vi "update_zc_info2A.vi"(0 "ywxinxi":string, 4 "didian":string, 5 "ruku":string, 6 "number":string, 7 "lingyong":string, 8 "syren":string, 9 "zrren":string, 10 "zrbumen":string) -> (1 "data_str":string)   [LabVIEW 2017, in "Lib_code.lvlib"]
uses:
  Lib_code.lvlib
panel:
  out "error":errorcluster caption="error out 4"
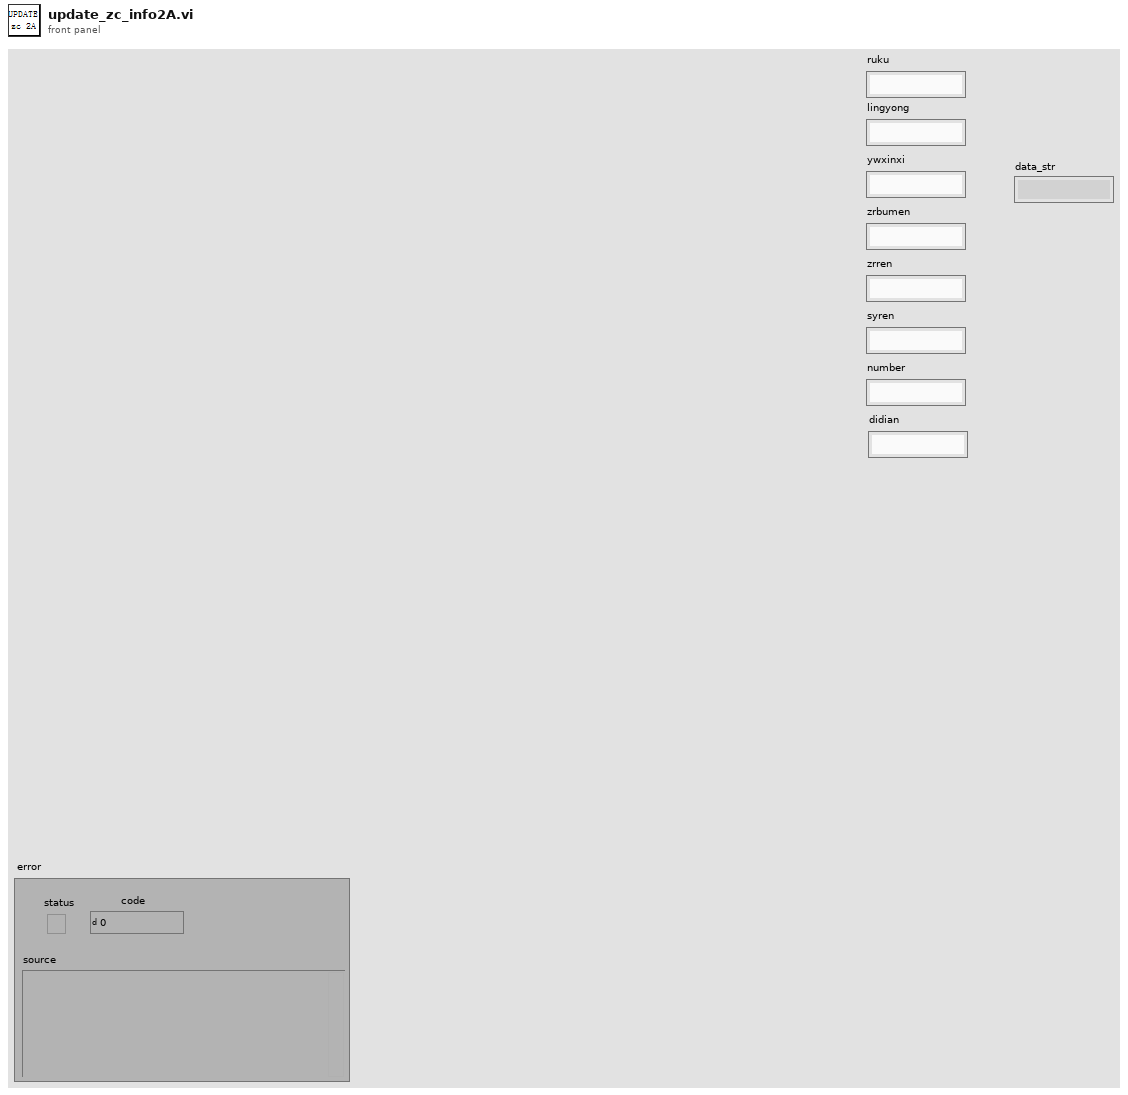
[diagram p1: front panel]
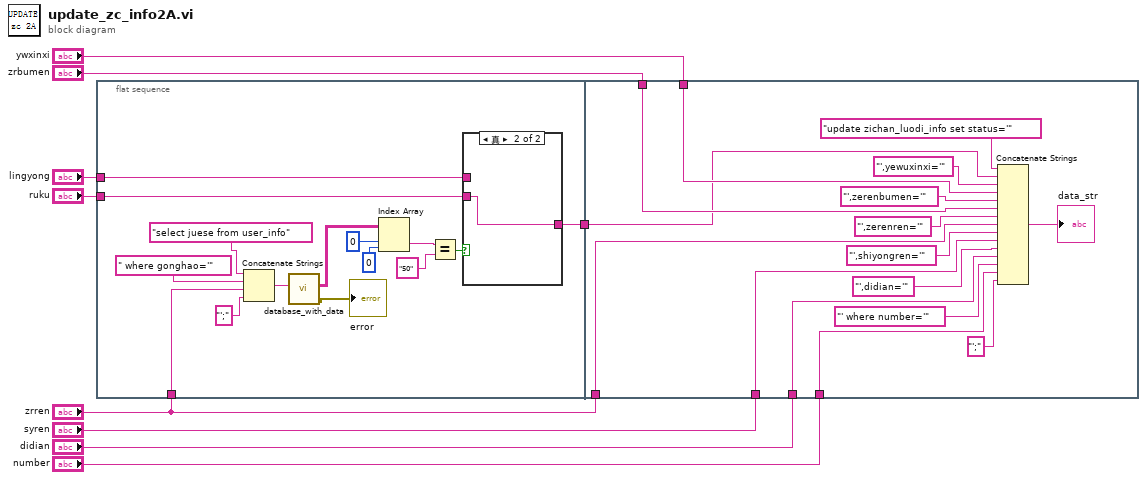
[diagram p0: block diagram]
diagram:
  n1 = flat-sequence {
    tunnel: "lingyong" -> [w13]
    tunnel: "ruku" -> [w12]
    tunnel: [w11] -> w2
    tunnel: "zrren" -> [w10]
    tunnel: "zrbumen" -> [w33]
    tunnel: "ywxinxi" -> [w32]
    tunnel: "didian" -> [w31]
    tunnel: "number" -> [w30]
    tunnel: "syren" -> [w29]
    tunnel: "zrren" -> [w28]
    tunnel: w2 -> [w27]
    frame #0 {
      n2 = Concatenate Strings("select juese from user_info" ("Command Text"), " where gonghao='" ("Command Text"), w10, "';" ("字符串")) -> (w20:string)
      n3 = call "database_with_data.vi"("input"=w20) -> ("error"=→"error":errorcluster, "Data"=w22:string[][])  [unwired: 9 in]
      n4 = Index Array(array=w22, index (row)=0 ("索引 (行)"), index (col)=0 ("禁用的索引 (列)")) -> (element=w23:string)
      n5 = Equal?(x=w23, y="50") -> (x = y?=w24:bool)
      n6 = case shown="真" w24 {
        tunnel: w13 -> [w25 _]
        tunnel: w12 -> [_ w26]
        tunnel: [w25 w26] -> w11
        frame False {
        }
        frame True {
        }
      }
    }
    frame #1 {
      n7 = Concatenate Strings("update zichan_luodi_info set status='" ("Command Text"), w27, "',yewuxinxi='" ("字符串"), w32, "',zerenbumen='" ("字符串"), w33, "',zerenren='" ("字符串"), w28, "',shiyongren='" ("字符串"), w29, "',didian='" ("字符串"), w31, "' where number='" ("字符串"), w30, "';" ("字符串")) -> (→"data_str":string)
    }
  }
